vi "CVT Static Reader.vi"(8 "error in (no error)":errorcluster) -> ()   [LabVIEW 2010]
panel:
  out "Waveform Chart 2":dbl(graph)
  out "Waveform Chart":i32(graph)
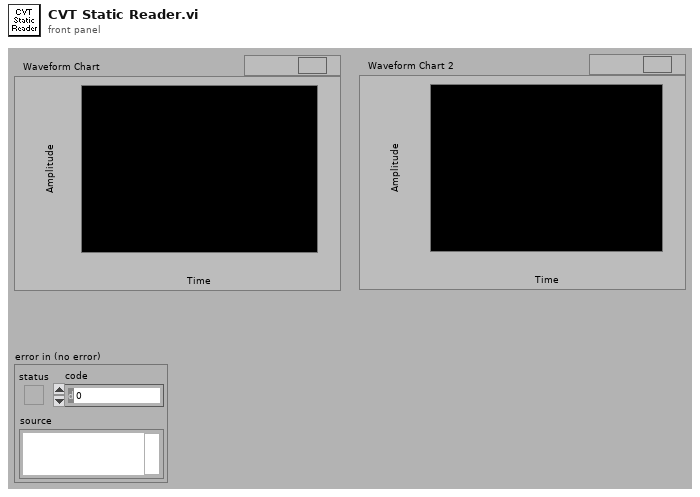
[diagram p1: front panel]
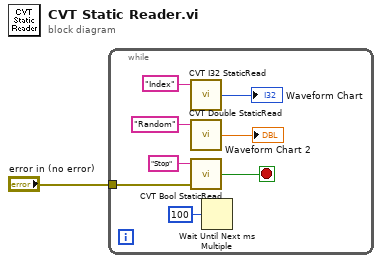
[diagram p0: block diagram]
diagram:
  n1 = while {
    tunnel: "error in (no error)" -> [w2]
    stop <- w4 stop-if-true
    n2 = call "CVT I32 StaticRead.vi"("Tag Name"="Index") -> ("Value"=→"Waveform Chart":i32)  [unwired: 1 in, 3 out]
    n3 = call "CVT Double StaticRead.vi"("Tag Name"="Random") -> ("Value"=→"Waveform Chart 2":dbl)  [unwired: 1 in, 3 out]
    n4 = call "CVT Bool StaticRead.vi"("error in (no error)"=w2, "Tag Name"="Stop") -> ("Value"=w4:bool)  [unwired: 3 out]
    n5 = Wait Until Next ms Multiple(millisecond multiple=u32 100) -> ()  [unwired: 1 out]
  }
